vi "VI Tree - time.vi"   [LabVIEW 2020]
panel:
  # "[OpenG VI Tags] ***Do Not Remove***"
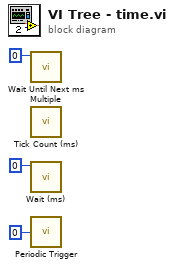
[diagram p0: block diagram]
diagram:
  n1 = call "Wait Until Next ms Multiple.vi"("milliseconds to wait"=u32 0) -> ()  [unwired: 9 in, 2 out]
  n2 = call "Tick Count (ms).vi"() -> ()  [unwired: 10 in, 2 out]
  n3 = call "Wait (ms).vi"("milliseconds to wait"=u32 0) -> ()  [unwired: 9 in, 2 out]
  n4 = call "Periodic Trigger.vi"("time (ms)"=u32 0) -> ()  [unwired: 12 in, 3 out]
